vi "zadanie_4_sinus.vi"() -> ()   [LabVIEW 2024]
panel:
  out "Waveform Graph":dbl[][](graph)
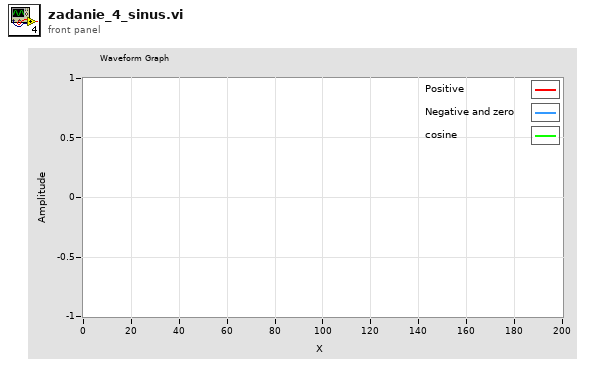
[diagram p1: front panel]
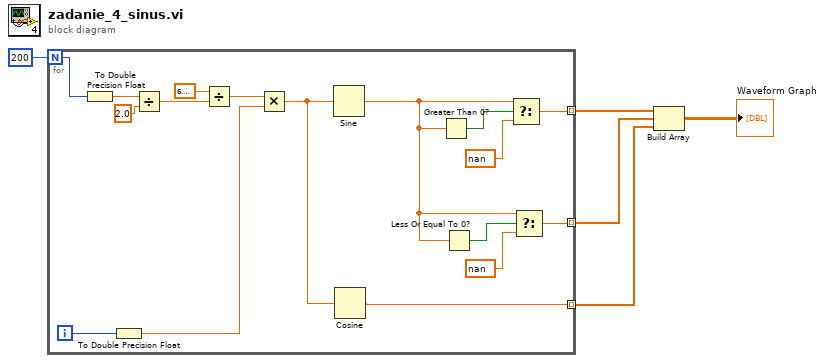
[diagram p0: block diagram]
diagram:
  n1 = for {
    N: 200 -> [w22]
    tunnel: [w17] -> w4 mode=indexing
    tunnel: [w9] -> w3 mode=indexing
    tunnel: [w6] -> w1 mode=indexing
    i -> [w19]
    n2 = To Double Precision Float(number=w22) -> (double precision float=w15:dbl)
    n3 = To Double Precision Float(number=w19) -> (double precision float=w18:dbl)
    n4 = Divide(x=w15, y=2.0) -> (x/y=w16:dbl)
    n5 = Divide(x=6.283185307179586, y=w16) -> (x/y=w20:dbl)
    n6 = Multiply(x=w20, y=w18) -> (x*y=w7:dbl)
    n7 = Sine(x=w7) -> (sin(x)=w8:dbl)
    n8 = Cosine(x=w7) -> (cos(x)=w6:dbl)
    n9 = Greater Than 0?(x=w8) -> (x > 0?=w13:bool)
    n10 = Less Or Equal To 0?(x=w8) -> (x <= 0?=w12:bool)
    n11 = Select(t=w8, s=w13, f=nan) -> (s? t:f=w17:dbl)
    n12 = Select(t=w8, s=w12, f=nan) -> (s? t:f=w9:dbl)
  }
  n13 = Build Array(w4, w3, w1) -> (→"Waveform Graph":dbl[][])
